vi "macrotoGFG.vi"() -> ()   [LabVIEW 2012]
uses:
  <vilib>/regexp/Match Regular Expression.xnode
panel:
  out "text":string
  out "Array 3":string[](array[string])
  in  "Path":path
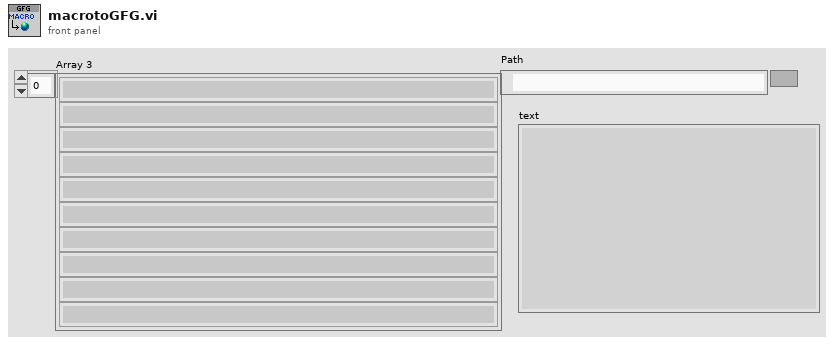
[diagram p1: front panel]
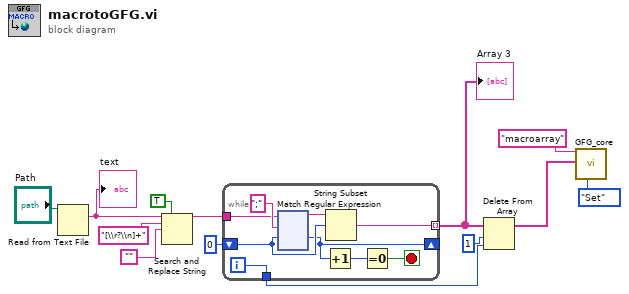
[diagram p0: block diagram]
diagram:
  n1 = Read from Text File(file (use dialog)="Path") -> (text=w11:string)  [unwired: 3 in, 3 out]
  "text" <- w11
  n2 = Search and Replace String(replace all?=TRUE ("replace all? (F)"), input string=w11, search string="[\\r?\\n]+", replace string="") -> (result string=w7:string)  [unwired: 4 in, 3 out]
  n3 = while {
    tunnel: w7 -> [w19]
    shift-right: [w15] -> _
    shift-left: 0 ("offset of match") -> [w16]
    tunnel: [w17] -> w6 mode=indexing
    tunnel: [w14] -> w5
    i -> [w14]
    stop <- w22 stop-if-true
    n4 = xnode "Match Regular Expression"("input string"=w19, "regular expression"=";" ("search string/char (-)"), "offset (0)"=w16) -> ("before match"=w18:string, "offset past match"=w15:i32)  [unwired: 3 in, 3 out]
    n5 = Increment(x=w15) -> (x+1=w21:i32)
    n6 = String Subset(string=w18, offset (0)=w16) -> (substring=w17:string)  [unwired: 1 in]
    n7 = Equal To 0?(x=w21) -> (x = 0?=w22:bool)
  }
  "Array 3" <- w6
  n8 = Delete From Array(array=w6, length=1, index=w5) -> (array with subset deleted=w2:string[])  [unwired: 1 out]
  n9 = call "GFG_core.vi"("Variable Name in"="macroarray", "Variant in"=w2, "Action"=enum16{"Init", "Set", "Get"}."Set") -> ()  [unwired: 10 in, 7 out]
